vi "RSZVB Set Power Coeficients.vi"(8 "error in (no error)":errorcluster {"code" format="%.0x"}, 9 "Coeficient":dbl[](array[numeric]) format="%^.3e", 10 "Port (1)":i32=1, 11 "VISA session":refnum<visa-resource-name>) -> (0 "error out":errorcluster {"code" format="%.0x"}, 3 "dup VISA session":refnum<visa-resource-name>)   [LabVIEW 2011]
doc: "Defines power coefficients for frequency converters R&S ZVA-ZxxxE. \n\nNotes:\n\n(1) This command is available for frequency converters with electronic attenuators R&S ZVA-ZxxxE.\n\nRemote-control command(s):\n[SENSe<Ch>:]FREQuency:CONVersion:DEVice:PCOefficient<Port> <C0>, <C1>, <C2>, <C3>"
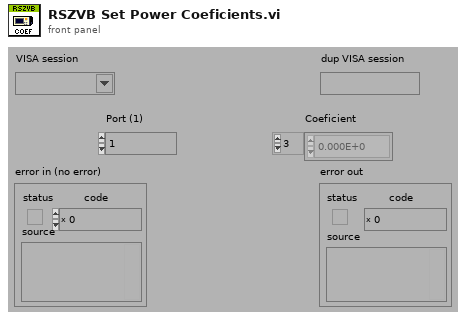
[diagram p1: front panel]
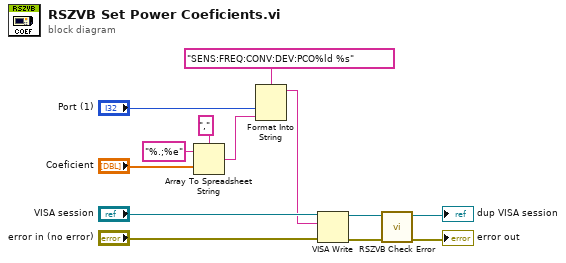
[diagram p0: block diagram]
diagram:
  n1 = Array To Spreadsheet String(delimiter (Tab)=",", array="Coeficient", 3:"%.;%e" ("format string")) -> (spreadsheet string=w8:string)
  n2 = Format Into String(format string="SENS:FREQ:CONV:DEV:PCO%ld %s", "Port (1)", w8) -> (resulting string=w5:string)  [unwired: 2 in, 1 out]
  n3 = VISA Write(VISA resource name="VISA session", write buffer=w5, error in (no error)="error in (no error)") -> (VISA resource name out=w3:refnum<visa-resource-name>, error out=w4:errorcluster)  [unwired: 1 out]
  n4 = call "RSZVB Check Error.vi"("error in (no error)"=w4, "VISA session"=w3) -> ("error out"=→"error out":errorcluster, "dup VISA session"=→"dup VISA session":refnum<visa-resource-name>)  [unwired: 8 in]
